vi "DER Randomize Measurements.vi"(10 "DeviceID":T2) -> (3 "DER Measurement Array":T1[](array[typedef]))   [LabVIEW 2018, in "IED Test Framework.lvlib" / "IED Test.lvclass"]
uses:
  IED Test.lvclass
  <vilib>/ORNL/CSEISMIC DDS/CSEISMIC DDS Base/Data Types/Controls/DeviceID.ctl
  <vilib>/ORNL/CSEISMIC DDS/CSEISMIC DDS Base/Data Types/DER_Measurement.ctl
  <vilib>/ORNL/CSEISMIC DDS/CSEISMIC DDS Base/CSEISMIC DDS.lvclass
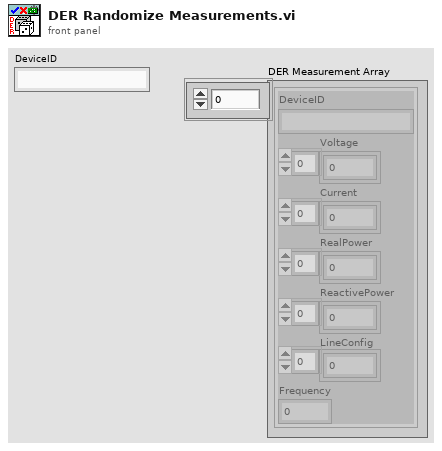
[diagram p1: front panel]
types:
  T1 = typedef "CSEISMIC DDS.lvlib/CSEISMIC DDS.lvclass/DER_Measurement.ctl" = cluster{"DeviceID":T2, "Voltage":dbl[], "Current":dbl[], "RealPower":dbl[], "ReactivePower":dbl[], "LineConfig":u8[], "Frequency":dbl}
  T2 = typedef "CSEISMIC DDS.lvlib/CSEISMIC DDS.lvclass/DeviceID.ctl" = string
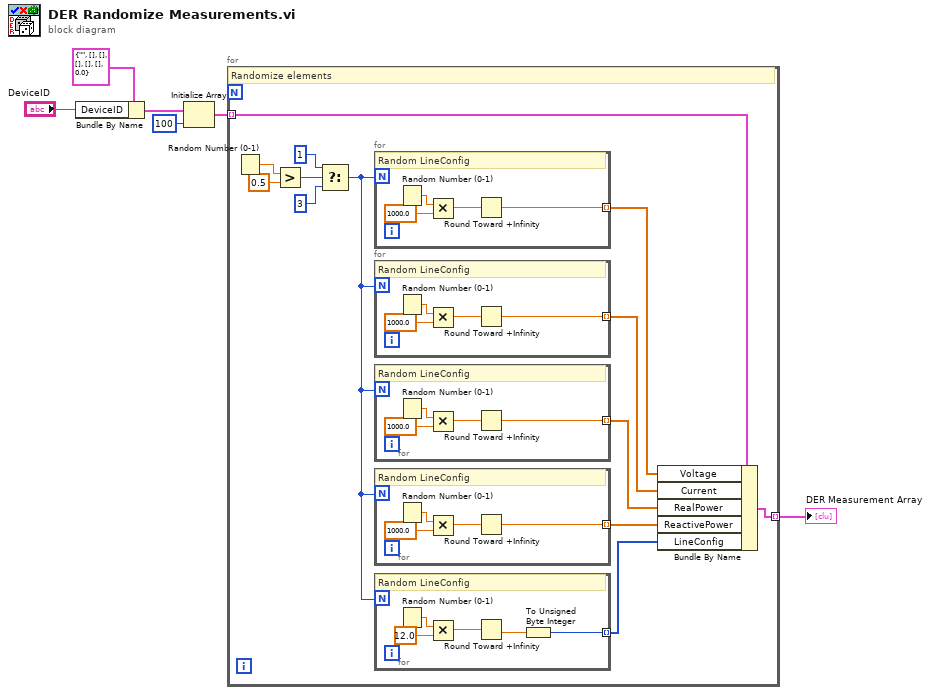
[diagram p0: block diagram]
diagram:
  n1 = Bundle By Name(cluster=T1 {"DeviceID"="", "Voltage"=[], "Current"=[], "RealPower"=[], "ReactivePower"=[], "LineConfig"=[], "Frequency"=0.0} ("DER_Measurement"), "DeviceID"="DeviceID") -> (w6:T1)
  n2 = Initialize Array(w6, 100 ("dimension size")) -> (w3:T1[])
  n3 = for {
    tunnel: w3 -> [w19] mode=indexing
    tunnel: [w18] -> w1 mode=indexing
    # "Randomize elements"
    n4 = Random Number (0-1)() -> (number: 0 to 1=w16:dbl)
    n5 = Greater?(x=w16, y=0.5) -> (0:w15:bool)
    n6 = Select(t=1, s=w15, f=3) -> (s? t:f=w7:i32)
    n7 = for {
      N: w7 -> [_]
      tunnel: [w37] -> w11 mode=indexing
      # "Random LineConfig"
      n8 = Random Number (0-1)() -> (number: 0 to 1=w40:dbl)
      n9 = Multiply(x=w40, y=1000.0) -> (x*y=w38:dbl)
      n10 = Round Toward +Infinity(x=w38) -> (ceil(x): smallest int >= x=w37:dbl)
    }
    n11 = for {
      N: w7 -> [_]
      tunnel: [w28] -> w10 mode=indexing
      # "Random LineConfig"
      n12 = Random Number (0-1)() -> (number: 0 to 1=w31:dbl)
      n13 = Multiply(x=w31, y=1000.0) -> (x*y=w29:dbl)
      n14 = Round Toward +Infinity(x=w29) -> (ceil(x): smallest int >= x=w28:dbl)
    }
    n15 = for {
      N: w7 -> [_]
      tunnel: [w24] -> w9 mode=indexing
      # "Random LineConfig"
      n16 = Random Number (0-1)() -> (number: 0 to 1=w27:dbl)
      n17 = Multiply(x=w27, y=1000.0) -> (x*y=w25:dbl)
      n18 = Round Toward +Infinity(x=w25) -> (ceil(x): smallest int >= x=w24:dbl)
    }
    n19 = for {
      N: w7 -> [_]
      tunnel: [w20] -> w8 mode=indexing
      # "Random LineConfig"
      n20 = Random Number (0-1)() -> (number: 0 to 1=w23:dbl)
      n21 = Multiply(x=w23, y=1000.0) -> (x*y=w21:dbl)
      n22 = Round Toward +Infinity(x=w21) -> (ceil(x): smallest int >= x=w20:dbl)
    }
    n23 = for {
      N: w7 -> [_]
      tunnel: [w32] -> w12 mode=indexing
      # "Random LineConfig"
      n24 = Random Number (0-1)() -> (number: 0 to 1=w36:dbl)
      n25 = Multiply(x=w36, y=12.0) -> (x*y=w34:dbl)
      n26 = Round Toward +Infinity(x=w34) -> (ceil(x): smallest int >= x=w33:dbl)
      n27 = To Unsigned Byte Integer(number=w33) -> (unsigned 8bit integer=w32:u8)
    }
    n28 = Bundle By Name(cluster=w19, "Voltage"=w11, "Current"=w10, "RealPower"=w9, "ReactivePower"=w8, "LineConfig"=w12) -> (w18:T1)
  }
  "DER Measurement Array" <- w1
